vi "LimitStatus.vi"(0 "VisaCluster":T1, 11 "error in (no error)":errorcluster) -> (4 "VisaCluster":T1, 8 "Answer":string, 10 "Limit":bool, 15 "error out":errorcluster)   [LabVIEW 2014, in "FH 55.lvlib"]
doc: "Dieses VI zeigt ob die LIMIT-Funktion eingeschaltet oder ausgeschaltet ist.\n\nThis VI shows whether the LIMIT function is turned on or off."
uses:
  FH 55.lvlib
  TypeDef/VisaCluster.ctl
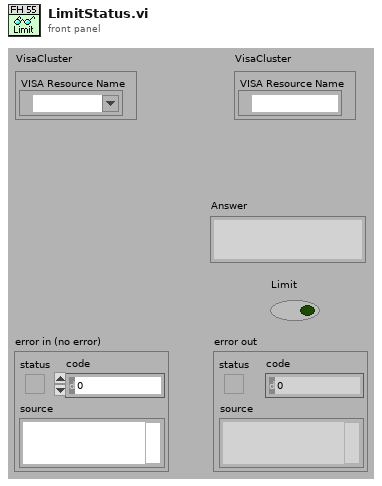
[diagram p1: front panel]
types:
  T1 = typedef "FH 55.lvlib/VisaCluster.ctl" = cluster{"VISA Resource Name":refnum<visa-resource-name>}
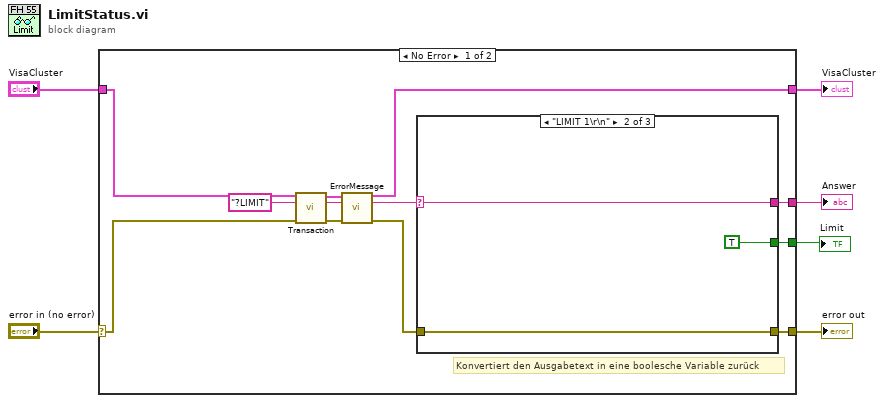
[diagram p0: block diagram]
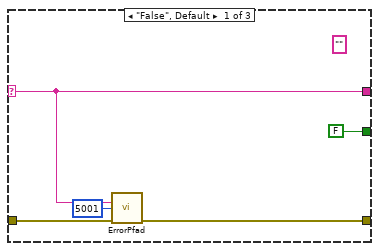
[diagram p2: hidden frame]
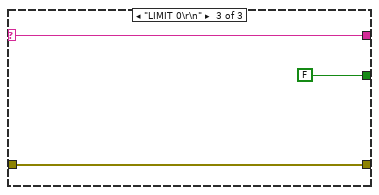
[diagram p3: hidden frame]
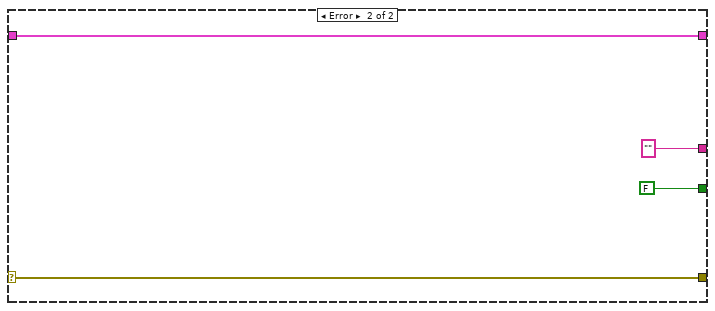
[diagram p4: hidden frame]
diagram:
  n1 = case shown="No Error" "error in (no error)" {
    selector: "error in (no error)" -> [w7 w32]
    tunnel: "VisaCluster" -> [w8 w33]
    tunnel: [w18 w33] -> w2
    tunnel: [w12 w32] -> w4
    tunnel: [w11 ""] -> w3
    tunnel: [w14 FALSE] -> w1
    frame No Error {
      # "Konvertiert den Ausgabetext in eine boolesche Variable zurück"
      n2 = call "Transaction.vi"("VisaCluster"=w8, "Command"="?LIMIT", "error in (no error)"=w7) -> ("VisaCluster"=w16:T1, "Answer"=w9:string, "error out"=w17:errorcluster)  [unwired: 9 in, 1 out]
      n3 = call "ErrorMessage.vi"("VisaCluster"=w16, "Message In"=w9, "error in (no error)"=w17) -> ("VisaCluster"=w18:T1, "Message Out"=w10:string, "error out"=w13:errorcluster)  [unwired: 10 in]
      n4 = case shown="\"LIMIT 1\\r\\n\"" w10 {
        selector: w10 -> [w19 w24 w28]
        tunnel: [FALSE TRUE FALSE] -> w14
        tunnel: w13 -> [w22 w25 w27]
        tunnel: [w21 w25 w27] -> w12
        tunnel: [w19 w24 w28] -> w11
        frame "False", Default {
          (unwired) ""
          n5 = call "ErrorPfad.vi"("Message In"=w19, "Numeric"=5001, "error in (no error)"=w22) -> ("error out"=w21:errorcluster)  [unwired: 11 in, 1 out]
        }
        frame "LIMIT 1\r\n" {
        }
        frame "LIMIT 0\r\n" {
        }
      }
    }
    frame Error {
    }
  }
  "error out" <- w4
  "Answer" <- w3
  "VisaCluster" <- w2
  "Limit" <- w1
